vi "4461 - Create Reference Waveforms.vi"(6 "sampling info":cluster{"Fs":dbl, "#s":dbl}={"Fs"=1000.0, "#s"=1000.0} {"Fs" format="%.2p"}, 8 "error in (no error)":errorcluster, 10 "reset signal":bool, 11 "Lockin":T1={"REF f (Hz)"=[13.0, 13.0, 13.0, 13.0, 13.0, 13.0, 13.0, 13.0], "REF phi (°)"=[0.0, 0.0, 0.0, 0.0, 0.0, 0.0, 0.0, 0.0]} {"REF phi (°)" format="%#_3g"}) -> (0 "error out":errorcluster, 1 "phase out":dbl[](array[numeric]), 2 "REF Array":waveform(dbl)[](array[waveform]), 3 "Lockin 2":T1={"REF f (Hz)"=[13.0, 13.0, 13.0, 13.0, 13.0, 13.0, 13.0, 13.0], "REF phi (°)"=[0.0, 0.0, 0.0, 0.0, 0.0, 0.0, 0.0, 0.0]} {"REF phi (°)" format="%#_3g"})   [LabVIEW 2016, in "LockinDAQ.lvclass"]
uses:
  LockinDAQ.lvclass
  Typedefs/REF-cluster.ctl
  Typedefs/REF_f-array.ctl
  Typedefs/REF_phi-array.ctl
  <vilib>/measure/NI_MABase.lvlib
panel:
  out "Waveform Graph 2":waveform(dbl)[](graph)
  out "Numeric":i32
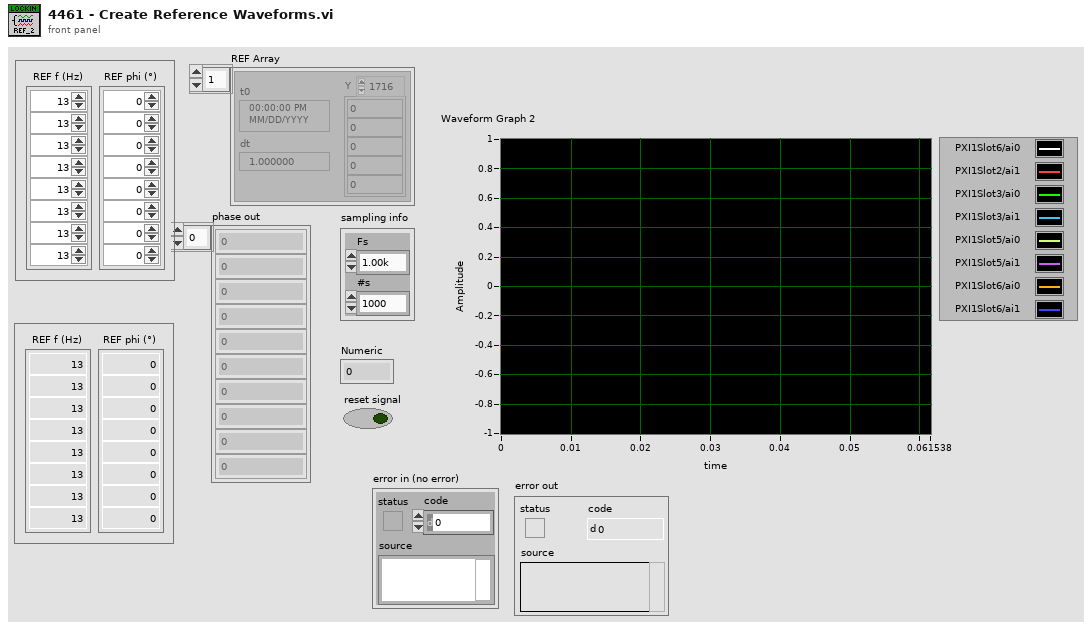
[diagram p1: front panel]
types:
  T1 = typedef "REF-cluster.ctl" = cluster{"REF f (Hz)":T2, "REF phi (°)":T3}
  T2 = typedef "REF_f-array.ctl" = dbl[]
  T3 = typedef "REF_phi-array.ctl" = dbl[]
  T4 = enum16{"Sine Wave", "Triangle Wave", "Square Wave", "Sawtooth Wave"}
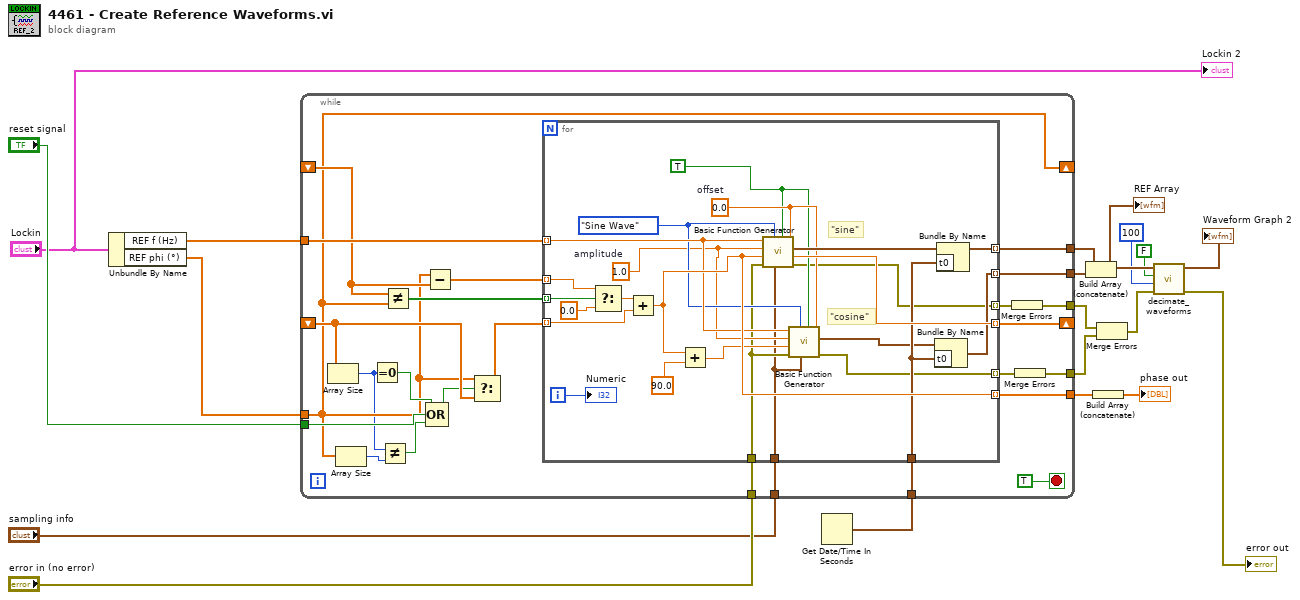
[diagram p0: block diagram]
diagram:
  n1 = Unbundle By Name("Lockin") -> ("REF f (Hz)"=w14:T2, "REF phi (°)"=w4:T3)
  n2 = Get Date/Time In Seconds() -> (seconds since 1Jan1904=w5:timestamp)
  n3 = while {
    tunnel: "sampling info" -> [w44]
    tunnel: [w43] -> w15
    tunnel: w4 -> [w23]
    tunnel: w14 -> [w42]
    shift-right: [w23] -> _
    shift-left: _ -> [w39]
    shift-right: [w37] -> _
    shift-left: _ -> [w34]
    tunnel: w5 -> [w35]
    tunnel: "reset signal" -> [w24]
    tunnel: [w31] -> w18
    tunnel: [w30] -> w16
    tunnel: "error in (no error)" -> [w29]
    tunnel: [w27] -> w8
    tunnel: [w25] -> w9
    stop <- TRUE stop-if-true
    n4 = Array Size(array=w34) -> (size(s)=w22:i32)
    n5 = Array Size(array=w23) -> (size(s)=w21:i32)
    n6 = Equal To 0?(x=w22) -> (x = 0?=w32:bool)
    n7 = Not Equal?(x=w22, y=w21) -> (x != y?=w20:bool)
    n8 = Not Equal?(x=w39, y=w23) -> (x != y?=w40:bool[])
    n9 = Subtract(x=w23, y=w39) -> (x-y=w38:T3)
    n10 = Compound Arithmetic op=OR(w32, w24, w20) -> (w33:bool)
    n11 = Select(t=w23, s=w33, f=w34) -> (s? t:f=w36:T3)
    n12 = for {
      tunnel: w42 -> [w56] mode=indexing
      tunnel: [w67] -> w43 mode=indexing
      tunnel: w44 -> [w47]
      tunnel: w40 -> [w61] mode=indexing
      tunnel: w38 -> [w63] mode=indexing
      tunnel: [w59] -> w37 mode=indexing
      tunnel: w36 -> [w64] mode=indexing
      tunnel: w35 -> [w55]
      tunnel: [w58] -> w31 mode=indexing
      tunnel: [w53] -> w30 mode=indexing
      tunnel: w29 -> [w48]
      tunnel: [w46] -> w28 mode=indexing
      tunnel: [w45] -> w26 mode=indexing
      i -> [w60]
      w49 = TRUE ("reset signal")
      w51 = 0.0  # offset
      w52 = T4."Sine Wave" ("signal type")
      w50 = 1.0  # amplitude
      # "\"cosine\""
      # "\"sine\""
      n13 = Select(t=w63, s=w61, f=0.0) -> (s? t:f=w65:dbl)
      n14 = Add(x=w65, y=w64) -> (x+y=w58:dbl)
      n15 = Add(x=w58, y=90.0) -> (x+y=w57:dbl)
      n16 = call <vilib>:"Basic Function Generator.vi"("offset"=w51, "reset signal"=w49, "sampling info"=w47, "signal type"=w52, "error in (no error)"=w48, "phase"=w58, "amplitude"=w50, "frequency"=w56) -> ("error out"=w46:errorcluster, "phase out"=w59:dbl, "signal out"=w68:waveform(dbl))  [unwired: 1 in]
      n17 = call <vilib>:"Basic Function Generator.vi"("offset"=w51, "reset signal"=w49, "sampling info"=w47, "signal type"=w52, "error in (no error)"=w48, "phase"=w57, "amplitude"=w50, "frequency"=w56) -> ("error out"=w45:errorcluster, "signal out"=w54:waveform(dbl))  [unwired: 1 in, 1 out]
      n18 = Bundle By Name(cluster=w54, "t0"=w55) -> (w53:waveform(dbl))
      n19 = Bundle By Name(cluster=w68, "t0"=w55) -> (w67:waveform(dbl))
      "Numeric" <- w60
    }
    n20 = Merge Errors(w28) -> (w27:errorcluster)
    n21 = Merge Errors(w26) -> (w25:errorcluster)
  }
  n22 = Build Array (concatenate)(w15, w16) -> (w11:waveform(dbl)[])
  "REF Array" <- w11
  n23 = Build Array (concatenate)(w18) -> (→"phase out":dbl[])
  n24 = Merge Errors(w8, w9) -> (w7:errorcluster)
  n25 = call "decimate_waveforms.vi"("Input Signal"=w11, "averaging"=FALSE, "decimating factor"=100, "error in (no error)"=w7) -> ("Decimated Waveforms"=→"Waveform Graph 2":waveform(dbl)[], "error out"=→"error out":errorcluster)  [unwired: 5 in]
  "Lockin 2" <- "Lockin"
